vi "Read fpgaVIRefCRIO9074.vi"(8 "error in (no error)":errorcluster, 11 "ComponentData in":refnum<class "ComponentData.lvclass">) -> (0 "error out":errorcluster, 2 "fpgaVIRefCRIO9074":T1, 3 "ComponentData out":refnum<class "ComponentData.lvclass">)   [LabVIEW 2013, in "ComponentData.lvlib" / "ComponentData.lvclass"]
uses:
  <userlib>/Common/Component/common_application/RT/ComponentData/ComponentData/ComponentData.lvclass
  <userlib>/Common/Component/common_application/RT/ComponentData/ComponentData/fpgaVIRefCRIO9074.ctl
  <userlib>/Common/Component/common_application/RT/ComponentData/ComponentData/ComponentData.lvclass/ComponentData.ctl
  <userlib>/Common/Component/common_application/RT/ComponentData.lvlib
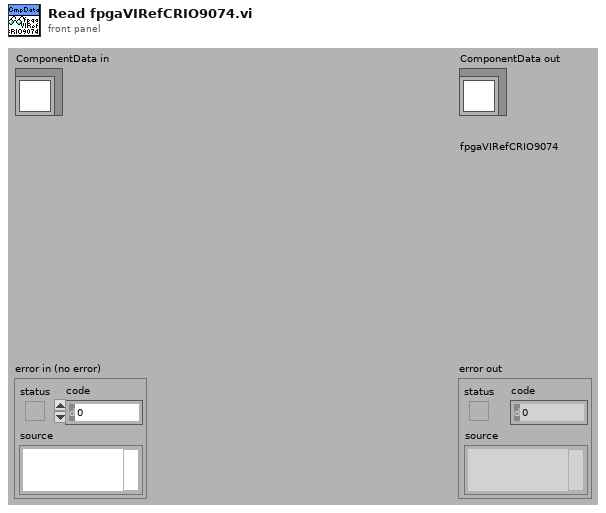
[diagram p1: front panel]
types:
  T1 = typedef "ComponentData.lvlib/fpgaVIRefCRIO9074.ctl" = refnum<k20>
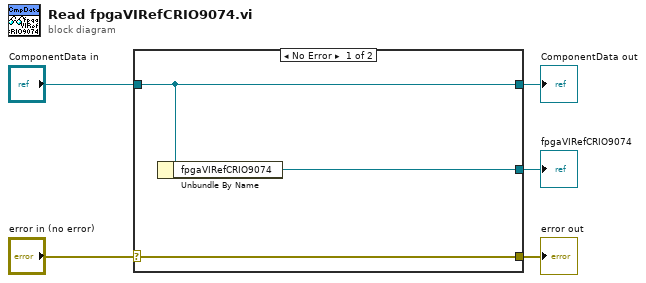
[diagram p0: block diagram]
diagram:
  n1 = case shown="No Error" "error in (no error)" {
    selector: "error in (no error)" -> [w8 w9]
    tunnel: [w8 w9] -> w4
    tunnel: [w7 w10] -> w2
    tunnel: "ComponentData in" -> [w7 w10]
    tunnel: [w6 _] -> w1
    frame No Error {
      n2 = Unbundle By Name(w7) -> ("fpgaVIRefCRIO9074"=w6:T1)
    }
    frame Error {
    }
  }
  "error out" <- w4
  "ComponentData out" <- w2
  "fpgaVIRefCRIO9074" <- w1
